vi "XIPIN_System_Cache_3_1.vi"   [LabVIEW 2017]
doc: "Multi-ported system cache connecting a Memory Controller with MicroBlaze and other AXI masters\n------------------------------------\n<b>Need License</b> : No\n<b>Interface</b> : AXI4"
uses:
  <vilib>/rvi/XilinxIP/XIPIN_XNode/niFpgaXIPIN.xnode
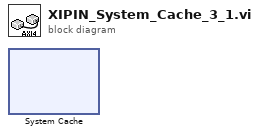
[diagram p0: block diagram]
diagram:
  n1 = xnode ("System Cache")() -> ()
